vi "Solicitar Contabilidad.vi"() -> ()   [LabVIEW 2020, in "UI.lvlib"]
uses:
  UI.lvlib
panel:
  in  "Solicitar":bool
  in  "Fecha Final":timestamp
  in  "Fecha Inicio":timestamp
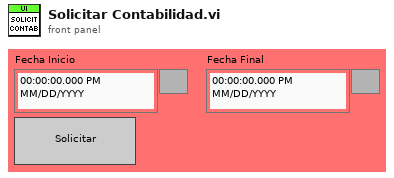
[diagram p1: front panel]
types:
  T1 = enum32{"Invalid", "Standard", "Closed", "Hidden", "Minimized", "Maximized"}
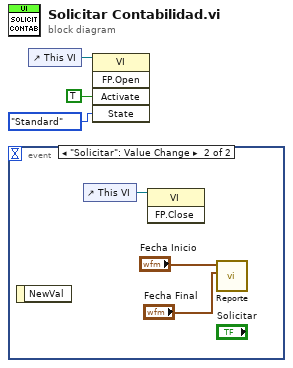
[diagram p0: block diagram]
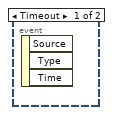
[diagram p2: hidden frame]
diagram:
  n1 = event shown="[1] \"Solicitar\": Value Change" {
    selector: _ -> [_ _]
    dyn-events: _ -> [_ _]
    timeout: _ -> [_ _]
    event Timeout {
      n2 = event-data() -> ()  [unwired: 1 in, 3 out]
    }
    event "Solicitar": Value Change {
      n3 = event-data() -> ()  [unwired: 1 in, 1 out]
      n4 = control-ref of="This VI"() -> (w6:refnum<vi>)
      n5 = invoke class="VI" method="FP.Close"(reference=w6) -> ()  [unwired: 2 in, 3 out]
      n6 = call "Reporte.vi"("End Time"="Fecha Final", "Start Time"="Fecha Inicio") -> ()  [unwired: 10 in]
    }
  }
  n7 = control-ref of="This VI"() -> (w1:refnum<vi>)
  n8 = invoke class="VI" method="FP.Open"(reference=w1, "Activate"=TRUE ("Activate?"), "State"=T1."Standard") -> ()  [unwired: 2 in, 5 out]
